vi "Baidu_Map_GET_Work.vi"() -> ()   [LabVIEW 2013]
uses:
  <vilib>/httpClient/LabVIEWHTTPClient.lvlib
panel:
  out "distance 2":string
  out "duration 2":string
  out "tollfee 2":string
  out "toll_distance 2":string
  out "minute 2":dbl
  out "hour 2":dbl
  out "error out 2":errorcluster
  in  "stop 2":bool
  out "loops 2":i32
  out "loops":i32
  in  "stop":bool
  out "error out":errorcluster
  out "hour":dbl
  out "minute":dbl
  out "toll_distance":string
  out "tollfee":string
  out "duration":string
  out "distance":string
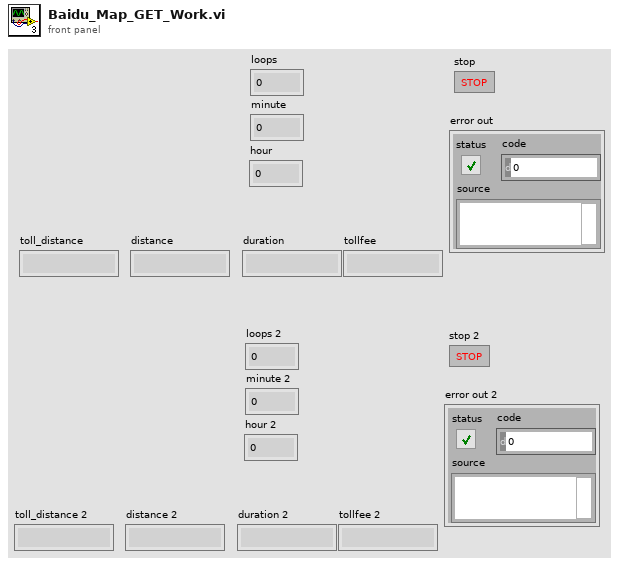
[diagram p1: front panel]
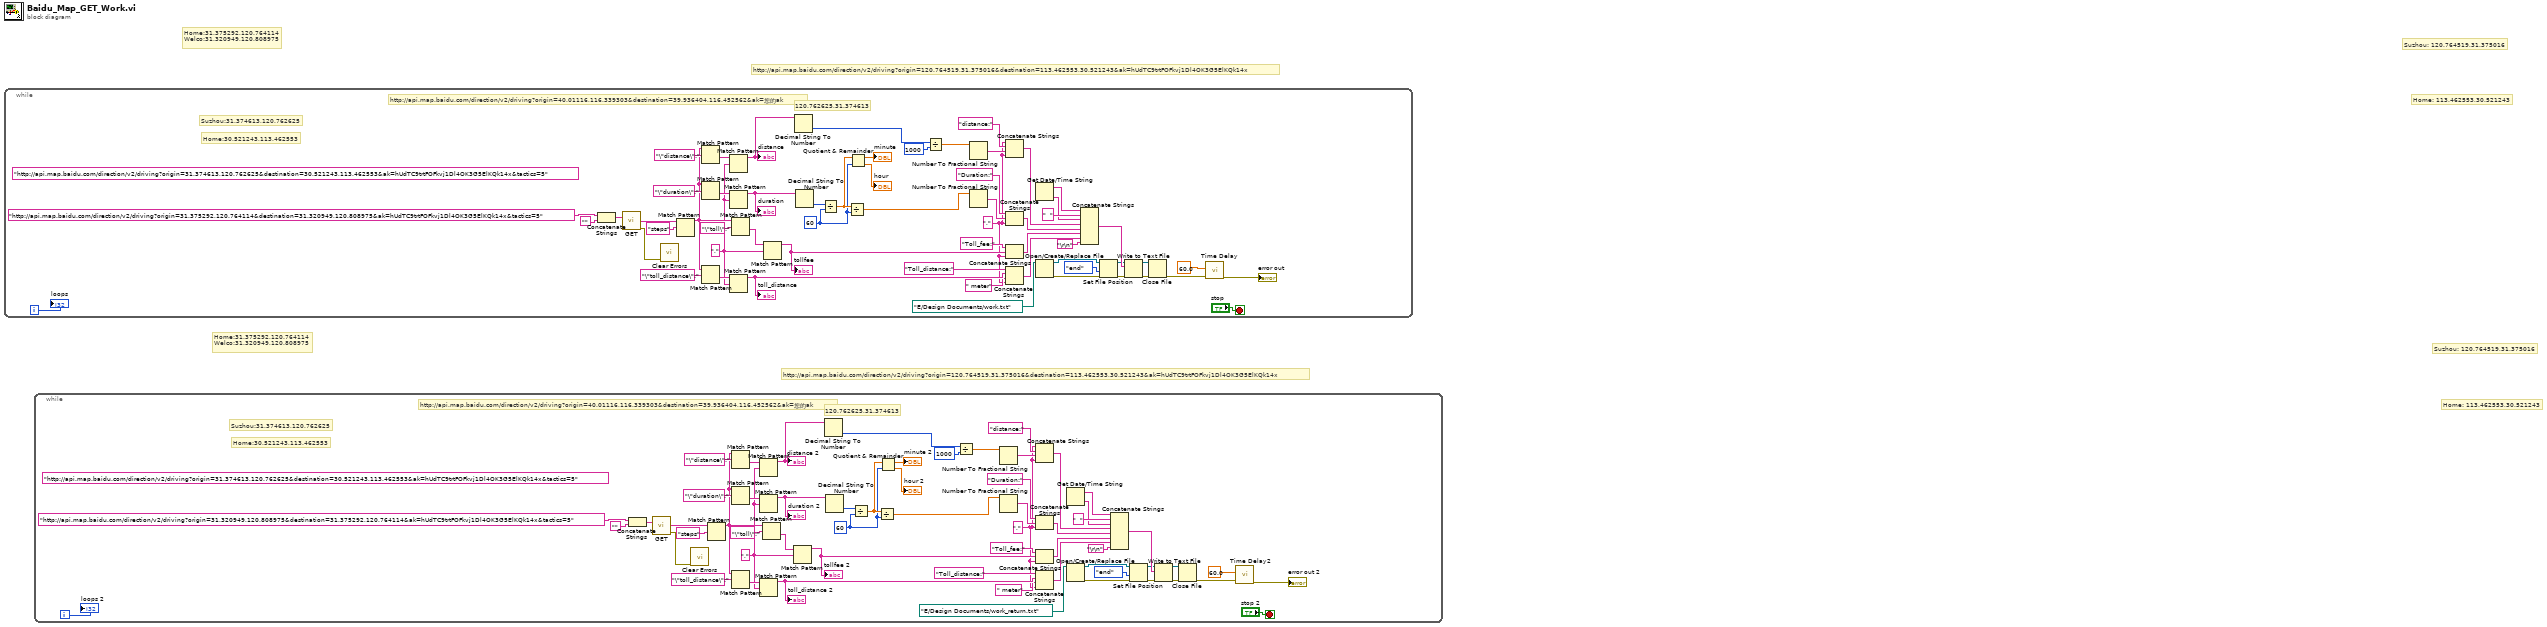
[diagram p0: block diagram]
diagram:
  # "Home:31.375292,120.764114\nWelco:31.320949,120.808975"
  # "http://api.map.baidu.com/direction/v2/driving?origin=40.01116,116.339303&destination=39.936404,116.452562&ak=您的ak"
  # "Home: 113.462553,30.521243"
  # "Suzhou: 120.764519,31.375016"
  # "http://api.map.baidu.com/direction/v2/driving?origin=120.764519,31.375016&destination=113.462553,30.521243&ak=hUdTC9trtFOFkvj1Dl4OK3G5ElKQk14x"
  # "Home:31.375292,120.764114\nWelco:31.320949,120.808975"
  # "http://api.map.baidu.com/direction/v2/driving?origin=40.01116,116.339303&destination=39.936404,116.452562&ak=您的ak"
  # "Home: 113.462553,30.521243"
  # "Suzhou: 120.764519,31.375016"
  # "http://api.map.baidu.com/direction/v2/driving?origin=120.764519,31.375016&destination=113.462553,30.521243&ak=hUdTC9trtFOFkvj1Dl4OK3G5ElKQk14x"
  n1 = while {
    i -> [w3]
    stop <- "stop" stop-if-true
    (unwired) "http://api.map.baidu.com/direction/v2/driving?origin=31.374613,120.762625&destination=30.521243,113.462553&ak=hUdTC9trtFOFkvj1Dl4OK3G5ElKQk14x&tactics=5" ("string")
    w22 = "," ("regular expression")
    w31 = 60 ("y")
    w47 = "," ("regular expression")
    # "Home:30.521243,113.462553"
    # "Suzhou:31.374613,120.762625"
    # "120.762625,31.374613"
    n2 = Concatenate Strings("http://api.map.baidu.com/direction/v2/driving?origin=31.375292,120.764114&destination=31.320949,120.808975&ak=hUdTC9trtFOFkvj1Dl4OK3G5ElKQk14x&tactics=5" ("string"), "") -> (w59:string)
    n3 = call <vilib>:"GET.vi"("url"=w59) -> ("body"=w8:string, "error out"=w2:errorcluster)  [unwired: 11 in, 2 out]
    n4 = call <vilib>:"Clear Errors.vi"("error in (no error)"=w2) -> ()  [unwired: 6 in, 1 out]
    n5 = Match Pattern(string=w8, regular expression="steps") -> (before substring=w49:string)  [unwired: 1 in, 3 out]
    n6 = Match Pattern(string=w49, regular expression="\"distance\":") -> (after substring=w55:string)  [unwired: 1 in, 3 out]
    n7 = Match Pattern(string=w49, regular expression="\"duration\":") -> (after substring=w53:string)  [unwired: 1 in, 3 out]
    n8 = Match Pattern(string=w49, regular expression="\"toll_distance\":") -> (after substring=w48:string)  [unwired: 1 in, 3 out]
    n9 = Match Pattern(string=w55, regular expression=w47) -> (before substring=w39:string)  [unwired: 1 in, 3 out]
    "distance" <- w39
    n10 = Match Pattern(string=w53, regular expression=w47) -> (before substring=w46:string)  [unwired: 1 in, 3 out]
    "duration" <- w46
    n11 = Match Pattern(string=w48, regular expression=w47) -> (before substring=w24:string)  [unwired: 1 in, 3 out]
    "toll_distance" <- w24
    n12 = Match Pattern(string=w49, regular expression="\"toll\":") -> (after substring=w51:string)  [unwired: 1 in, 3 out]
    n13 = Match Pattern(string=w51, regular expression=w47) -> (before substring=w26:string)  [unwired: 1 in, 3 out]
    "tollfee" <- w26
    n14 = Decimal String To Number(string=w39) -> (number=w38:i32)  [unwired: 2 in, 1 out]
    n15 = Decimal String To Number(string=w46) -> (number=w45:i32)  [unwired: 2 in, 1 out]
    n16 = Divide(x=w45, y=w31) -> (x/y=w32:dbl)
    n17 = Divide(x=w32, y=w31) -> (x/y=w30:dbl)
    n18 = Quotient & Remainder(x=w32, y=w31) -> (x-y*floor(x/y)=→"minute":dbl, floor(x/y)=→"hour":dbl)
    n19 = Divide(x=w38, y=1000) -> (x/y=w36:dbl)
    n20 = Number To Fractional String(number=w36) -> (F-format string=w34:string)  [unwired: 3 in]
    n21 = Number To Fractional String(number=w30) -> (F-format string=w28:string)  [unwired: 3 in]
    n22 = Concatenate Strings(w22, "distance:" ("string"), w34, w22) -> (w33:string)
    n23 = Concatenate Strings("Duration:" ("string"), w28, w22) -> (w21:string)
    n24 = Concatenate Strings("Toll_fee:" ("string"), w26, w22) -> (w20:string)
    n25 = Concatenate Strings("Toll_distance:" ("string"), w24, " meter" ("string"), w22) -> (w19:string)
    n26 = Get Date/Time String() -> (date string=w42:string, time string=w40:string)  [unwired: 3 in]
    n27 = Open/Create/Replace File(file path (use dialog)=path "E:/Design Documents/work.txt") -> (refnum out=w15:refnum<file>, error out=w13:errorcluster)  [unwired: 5 in, 1 out]
    n28 = Concatenate Strings(w42, "  " ("string"), w40, w33, w21, w20, w19, "\r\n") -> (w16:string)
    n29 = Set File Position(refnum=w15, from (0:start)=enum16{"start", "end", "current"}."end", error in=w13) -> (refnum out=w14:refnum<file>, error out=w11:errorcluster)  [unwired: 1 in]
    n30 = Write to Text File(file (use dialog)=w14, text=w16, error in=w11) -> (refnum out=w10:refnum<file>, error out=w9:errorcluster)  [unwired: 1 in, 1 out]
    n31 = Close File(refnum=w10, error in=w9) -> (error out=w6:errorcluster)  [unwired: 1 out]
    n32 = call "Time Delay"("error in (no error)"=w6, "Delay Time (s)"=60.0) -> ("error out"=→"error out":errorcluster)  [unwired: 9 in]
    "loops" <- w3
  }
  n33 = while {
    i -> [w62]
    stop <- "stop 2" stop-if-true
    (unwired) "http://api.map.baidu.com/direction/v2/driving?origin=31.374613,120.762625&destination=30.521243,113.462553&ak=hUdTC9trtFOFkvj1Dl4OK3G5ElKQk14x&tactics=5" ("string")
    w81 = "," ("regular expression")
    w90 = 60 ("y")
    w106 = "," ("regular expression")
    # "Home:30.521243,113.462553"
    # "Suzhou:31.374613,120.762625"
    # "120.762625,31.374613"
    n34 = Concatenate Strings("http://api.map.baidu.com/direction/v2/driving?origin=31.320949,120.808975&destination=31.375292,120.764114&ak=hUdTC9trtFOFkvj1Dl4OK3G5ElKQk14x&tactics=5" ("string"), "") -> (w118:string)
    n35 = call <vilib>:"GET.vi"("url"=w118) -> ("body"=w67:string, "error out"=w61:errorcluster)  [unwired: 11 in, 2 out]
    n36 = call <vilib>:"Clear Errors.vi"("error in (no error)"=w61) -> ()  [unwired: 6 in, 1 out]
    n37 = Match Pattern(string=w67, regular expression="steps") -> (before substring=w108:string)  [unwired: 1 in, 3 out]
    n38 = Match Pattern(string=w108, regular expression="\"distance\":") -> (after substring=w114:string)  [unwired: 1 in, 3 out]
    n39 = Match Pattern(string=w108, regular expression="\"duration\":") -> (after substring=w112:string)  [unwired: 1 in, 3 out]
    n40 = Match Pattern(string=w108, regular expression="\"toll_distance\":") -> (after substring=w107:string)  [unwired: 1 in, 3 out]
    n41 = Match Pattern(string=w114, regular expression=w106) -> (before substring=w98:string)  [unwired: 1 in, 3 out]
    "distance 2" <- w98
    n42 = Match Pattern(string=w112, regular expression=w106) -> (before substring=w105:string)  [unwired: 1 in, 3 out]
    "duration 2" <- w105
    n43 = Match Pattern(string=w107, regular expression=w106) -> (before substring=w83:string)  [unwired: 1 in, 3 out]
    "toll_distance 2" <- w83
    n44 = Match Pattern(string=w108, regular expression="\"toll\":") -> (after substring=w110:string)  [unwired: 1 in, 3 out]
    n45 = Match Pattern(string=w110, regular expression=w106) -> (before substring=w85:string)  [unwired: 1 in, 3 out]
    "tollfee 2" <- w85
    n46 = Decimal String To Number(string=w98) -> (number=w97:i32)  [unwired: 2 in, 1 out]
    n47 = Decimal String To Number(string=w105) -> (number=w104:i32)  [unwired: 2 in, 1 out]
    n48 = Divide(x=w104, y=w90) -> (x/y=w91:dbl)
    n49 = Divide(x=w91, y=w90) -> (x/y=w89:dbl)
    n50 = Quotient & Remainder(x=w91, y=w90) -> (x-y*floor(x/y)=→"minute 2":dbl, floor(x/y)=→"hour 2":dbl)
    n51 = Divide(x=w97, y=1000) -> (x/y=w95:dbl)
    n52 = Number To Fractional String(number=w95) -> (F-format string=w93:string)  [unwired: 3 in]
    n53 = Number To Fractional String(number=w89) -> (F-format string=w87:string)  [unwired: 3 in]
    n54 = Concatenate Strings(w81, "distance:" ("string"), w93, w81) -> (w92:string)
    n55 = Concatenate Strings("Duration:" ("string"), w87, w81) -> (w80:string)
    n56 = Concatenate Strings("Toll_fee:" ("string"), w85, w81) -> (w79:string)
    n57 = Concatenate Strings("Toll_distance:" ("string"), w83, " meter" ("string"), w81) -> (w78:string)
    n58 = Get Date/Time String() -> (date string=w101:string, time string=w99:string)  [unwired: 3 in]
    n59 = Open/Create/Replace File(file path (use dialog)=path "E:/Design Documents/work_return.txt") -> (refnum out=w74:refnum<file>, error out=w72:errorcluster)  [unwired: 5 in, 1 out]
    n60 = Concatenate Strings(w101, "  " ("string"), w99, w92, w80, w79, w78, "\r\n") -> (w75:string)
    n61 = Set File Position(refnum=w74, from (0:start)=enum16{"start", "end", "current"}."end", error in=w72) -> (refnum out=w73:refnum<file>, error out=w70:errorcluster)  [unwired: 1 in]
    n62 = Write to Text File(file (use dialog)=w73, text=w75, error in=w70) -> (refnum out=w69:refnum<file>, error out=w68:errorcluster)  [unwired: 1 in, 1 out]
    n63 = Close File(refnum=w69, error in=w68) -> (error out=w65:errorcluster)  [unwired: 1 out]
    n64 = call "Time Delay2"("error in (no error)"=w65, "Delay Time (s)"=60.0) -> ("error out"=→"error out 2":errorcluster)  [unwired: 9 in]
    "loops 2" <- w62
  }
